vi "subCallConfigRx.vi"(0 "session handle":refnum<k15>, 5 "Rx Parameters":T1={"Rx IQ Sampling\nRate [s/sec]"=200000.0, "Rx\nFrequency [Hz]"=433920000.0, "Rx Gain [dB]"=0.0, "Rx Antenna"="RX2"} {"Rx Gain [dB]" format="%#.6p"; "Rx\nFrequency [Hz]" format="%#.6p"; "Rx IQ Sampling\nRate [s/sec]" format="%#.6p"}, 11 "error in":errorcluster) -> (4 "session handle out":refnum<k15>, 6 "Actual Rx Parameters":T1 {"Rx Gain [dB]" format="%#.6p"; "Rx\nFrequency [Hz]" format="%#.6p"; "Rx IQ Sampling\nRate [s/sec]" format="%#.6p"}, 15 "error out":errorcluster)   [LabVIEW 2010]
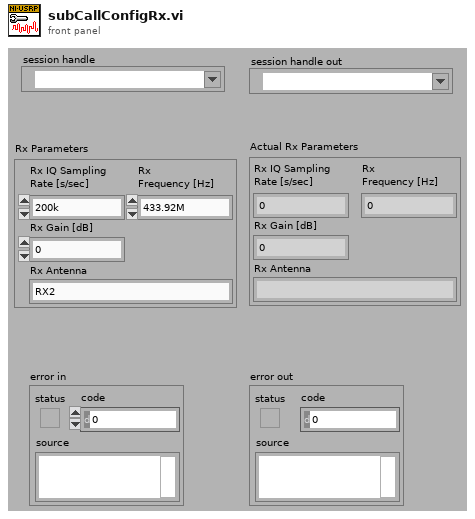
[diagram p1: front panel]
types:
  T1 = cluster{"Rx IQ Sampling\nRate [s/sec]":dbl, "Rx\nFrequency [Hz]":dbl, "Rx Gain [dB]":dbl, "Rx Antenna":string}
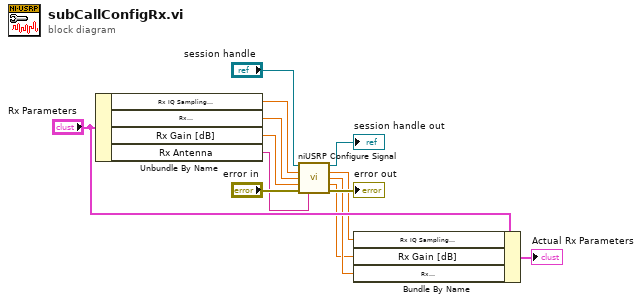
[diagram p0: block diagram]
diagram:
  n1 = Unbundle By Name("Rx Parameters") -> ("Rx IQ Sampling\nRate [s/sec]"=w7:dbl, "Rx\nFrequency [Hz]"=w8:dbl, "Rx Gain [dB]"=w9:dbl, "Rx Antenna"=w1:string)
  n2 = call <instrlib>:"niUSRP Configure Signal.vi"("session handle"="session handle", "IQ rate"=w7, "carrier frequency"=w8, "gain"=w9, "error in (no error)"="error in", "active antenna"=w1) -> ("session handle out"=→"session handle out":refnum<k15>, "coerced IQ rate"=w4:dbl, "coerced carrier frequency"=w3:dbl, "coerced gain"=w2:dbl, "error out"=→"error out":errorcluster)  [unwired: 5 in]
  n3 = Bundle By Name(cluster="Rx Parameters", "Rx IQ Sampling\nRate [s/sec]"=w4, "Rx Gain [dB]"=w2, "Rx\nFrequency [Hz]"=w3) -> (→"Actual Rx Parameters":T1)
